vi "Log Helper Action Errors and Warnings.vi"(8 "error in (no error)":errorcluster, 11 "Helper Loop in":refnum<class "Helper Loop.lvclass">) -> (0 "error out":errorcluster, 3 "Helper Loop Out":refnum<class "Helper Loop.lvclass">)   [LabVIEW 2020, in "Helper Loop.lvclass"]
uses:
  Helper Loop.lvclass
  Logging/Logging.lvclass
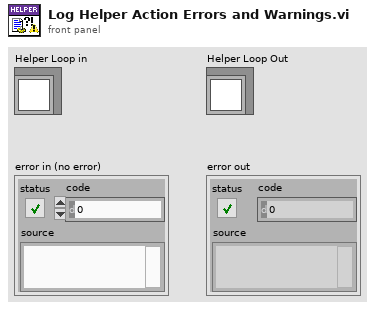
[diagram p1: front panel]
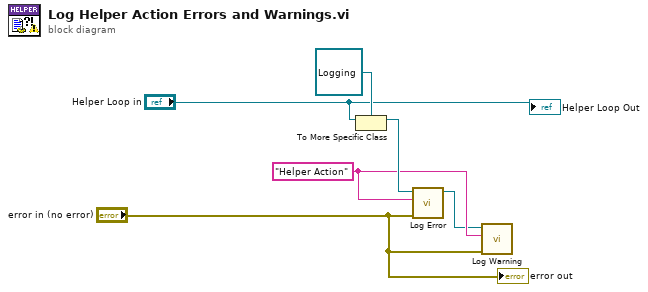
[diagram p0: block diagram]
diagram:
  w3 = "Helper Action" ("format string")
  n1 = To More Specific Class(target class=refnum<class "Logging.lvclass"> refnum ("Logging In"), reference="Helper Loop in") -> (specific class reference=w4:refnum<class "Logging.lvclass">)  [unwired: 1 in, 1 out]
  n2 = call "Log Error.vi"("error in (no error)"="error in (no error)", "Message"=w3, "Logging In"=w4) -> ("Logging Out"=w2:refnum<class "Logging.lvclass">)  [unwired: 7 in, 1 out]
  n3 = call "Log Warning.vi"("error in (no error)"="error in (no error)", "Message"=w3, "Logging In"=w2) -> ()  [unwired: 7 in, 2 out]
  "error out" <- "error in (no error)"
  "Helper Loop Out" <- "Helper Loop in"
